vi "Write Imaging Control.vi"(8 "error in (no error)":errorcluster, 10 "Imaging Control":refnum<k7>, 11 "IMG_SRC in":refnum<class "IMG_SRC.lvclass">) -> (0 "error out":errorcluster, 3 "IMG_SRC out":refnum<class "IMG_SRC.lvclass">)   [LabVIEW 2018, in "IMG_SRC.lvlib" / "IMG_SRC.lvclass"]
uses:
  IMG_SRC.lvclass
  IMG_SRC.lvclass/IMG_SRC.ctl
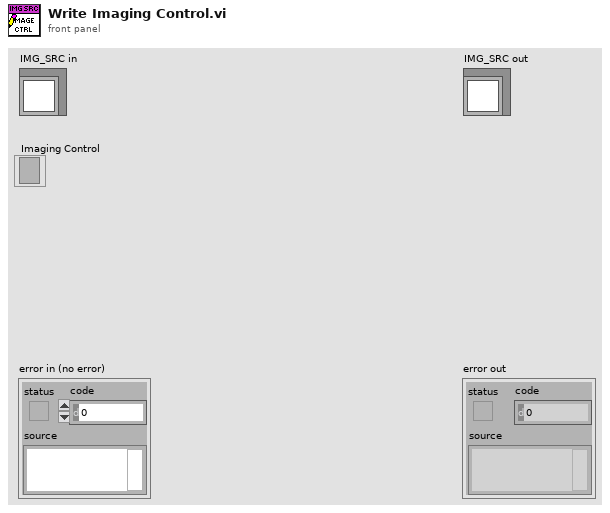
[diagram p1: front panel]
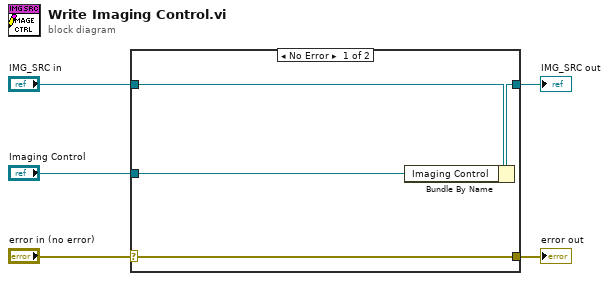
[diagram p0: block diagram]
diagram:
  n1 = case shown="No Error" "error in (no error)" {
    selector: "error in (no error)" -> [w9 w10]
    tunnel: [w9 w10] -> w4
    tunnel: [w7 w11] -> w2
    tunnel: "IMG_SRC in" -> [w8 w11]
    tunnel: "Imaging Control" -> [w6 _]
    frame No Error {
      n2 = Bundle By Name(cluster=w8, "Imaging Control"=w6) -> (w7:refnum<class "IMG_SRC.lvclass">)
    }
    frame Error {
    }
  }
  "error out" <- w4
  "IMG_SRC out" <- w2
